vi "RotateLogs.vi"(6 "max bytes (25000)":i32=25000, 7 "max log files (5)":i32=5, 8 "error in (no error)":errorcluster, 11 "log dir":path) -> (0 "error out":errorcluster)   [LabVIEW 2017, in "TraceLogger.lvlib"]
uses:
  <vilib>/addons/TraceLogger/TraceLogger.lvlib
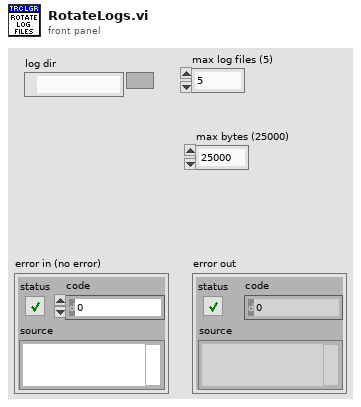
[diagram p1: front panel]
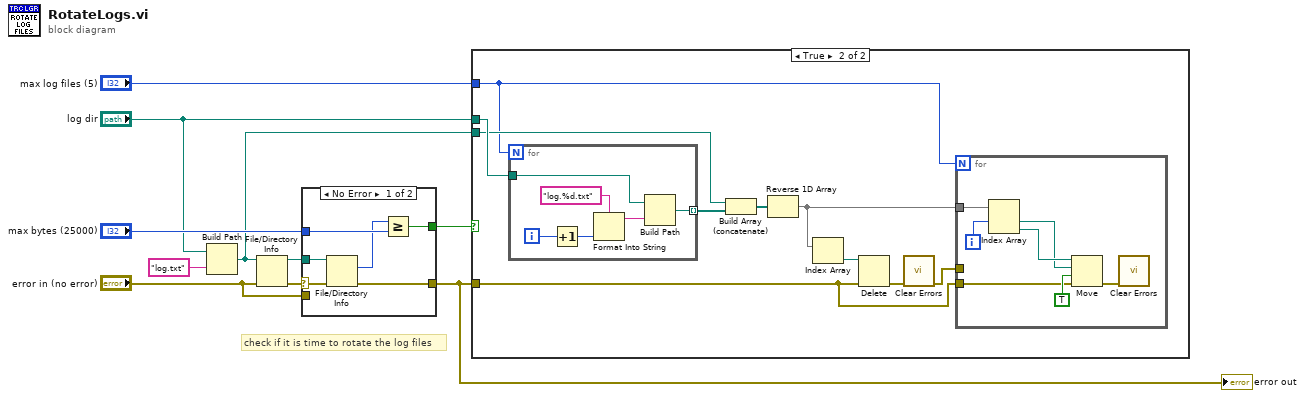
[diagram p0: block diagram]
diagram:
  # "check if it is time to rotate the log files"
  n1 = Build Path(base path="log dir", name or relative path="log.txt") -> (appended path=w2:path)
  n2 = File/Directory Info(path=w2, error in="error in (no error)") -> (path out=w8:path, error out=w7:errorcluster)  [unwired: 5 out]
  n3 = case shown="No Error" w7 {
    selector: w7 -> [w11 _]
    tunnel: "max bytes (25000)" -> [w16 _]
    tunnel: [w14 w17] -> w1
    tunnel: [w13 _] -> w5
    tunnel: w8 -> [w12 _]
    tunnel: "error in (no error)" -> [_ w17]
    frame No Error {
      n4 = File/Directory Info(path=w12, error in=w11) -> (size=w15:i64, error out=w14:errorcluster)  [unwired: 5 out]
      n5 = Greater Or Equal?(x=w15, y=w16) -> (x >= y?=w13:bool)
    }
    frame Error {
    }
  }
  "error out" <- w1
  n6 = case shown="True" w5 {
    tunnel: w1 -> [_ w19]
    tunnel: "max log files (5)" -> [_ w23]
    tunnel: "log dir" -> [_ w26]
    tunnel: w2 -> [_ w24]
    frame False {
    }
    frame True {
      n7 = for {
        N: w23 -> [_]
        tunnel: w26 -> [w29]
        tunnel: [w28] -> w25 mode=indexing
        i -> [w32]
        n8 = Increment(x=w32) -> (x+1=w31:i32)
        n9 = Format Into String(format string="log.%d.txt" ("name or relative path"), w31) -> (resulting string=w30:string)  [unwired: 2 in, 1 out]
        n10 = Build Path(base path=w29, name or relative path=w30) -> (appended path=w28:path)
      }
      n11 = Build Array (concatenate)(w24, w25) -> (w22:path[])
      n12 = Reverse 1D Array(array=w22) -> (reversed array=w20:path[])
      n13 = Index Array(array=w20) -> (element=w21:path)  [unwired: 1 in]
      n14 = Delete(path (use dialog)=w21, error in=w19) -> (error out=w27:errorcluster)  [unwired: 3 in, 2 out]
      n15 = call <vilib>:"Clear Errors.vi"("error in (no error)"=w27) -> ("error out"=w18:errorcluster)  [unwired: 5 in, 1 out]
      n16 = for {
        N: w23 -> [_]
        tunnel: w20 -> [w39]
        tunnel: w19 -> [w34]
        tunnel: w18 -> [_]
        i -> [w38]
        n17 = Index Array(array=w39, index #1=w38) -> (element #1=w35:path, element #2=w36:path)  [unwired: 1 in]
        n18 = Move(source path=w36, error in=w34, 9:TRUE ("overwrite (F)"), 10:w35) -> (error out=w37:errorcluster)  [unwired: 1 in, 2 out]
        n19 = call <vilib>:"Clear Errors.vi"("error in (no error)"=w37) -> ()  [unwired: 5 in, 2 out]
      }
    }
  }
